vi "recieving (SubVI).vi"(1 "TR":bool, 2 "TM":bool, 3 "TL":bool, 5 "CL":bool, 7 "CM":bool, 9 "CR":bool, 12 "BL":bool, 13 "BM":bool, 14 "BR":bool) -> (8 "appended array":dbl[](array[numeric]))   [LabVIEW 2009]
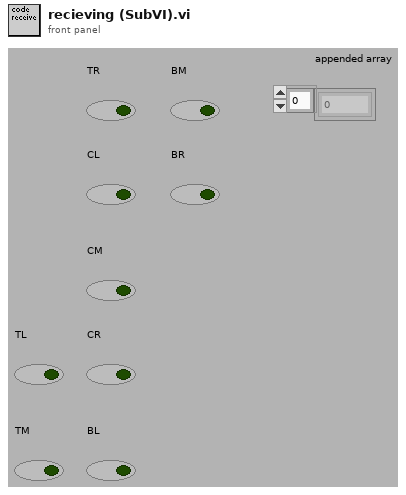
[diagram p1: front panel]
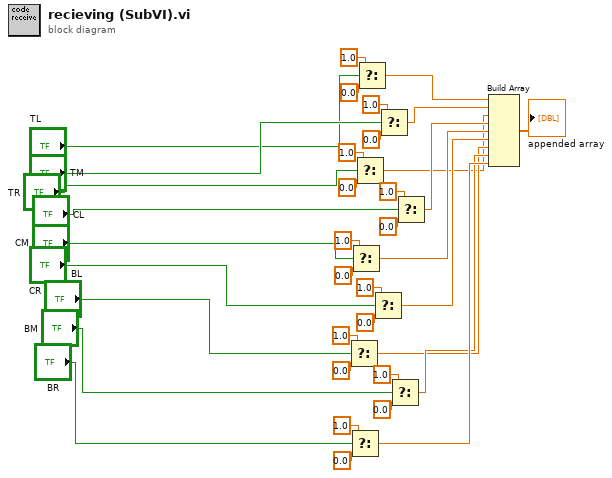
[diagram p0: block diagram]
diagram:
  n1 = Select(t=1.0, s="BL", f=0.0) -> (s? t:f=w34:dbl)
  n2 = Select(t=1.0, s="BR", f=0.0) -> (s? t:f=w36:dbl)
  n3 = Select(t=1.0, s="CM", f=0.0) -> (s? t:f=w32:dbl)
  n4 = Select(t=1.0, s="TR", f=0.0) -> (s? t:f=w30:dbl)
  n5 = Select(t=1.0, s="TL", f=0.0) -> (s? t:f=w28:dbl)
  n6 = Select(t=1.0, s="CR", f=0.0) -> (s? t:f=w33:dbl)
  n7 = Select(t=1.0, s="TM", f=0.0) -> (s? t:f=w29:dbl)
  n8 = Select(t=1.0, s="BM", f=0.0) -> (s? t:f=w35:dbl)
  n9 = Select(t=1.0, s="CL", f=0.0) -> (s? t:f=w31:dbl)
  n10 = Build Array(w28, w29, w30, w31, w32, w33, w34, w35, w36) -> (→"appended array":dbl[])
